vi "VSI Settings Dialog.vi"(8 "error in (no error)":errorcluster, 11 "Ctrl settings in":T1={"FSM status"=enum."Running", "Ctrl bypass"=FALSE, "PID Control"={"Ref_val"=0.0, "Kp"=0.0, "Ti"=0.0, "Td"=16.0, "Out_min"=0.0, "Out_max"=0.0}, "3rd Harmonic"=FALSE, "Output enable"=FALSE, "Phase DBG"=0}) -> (0 "error out":errorcluster, 1 "Cancelled?":bool, 2 "UI Refresh Needed?":bool, 3 "Ctrl settings out":T1={"FSM status"=enum."Running", "Ctrl bypass"=FALSE, "PID Control"={"Ref_val"=0.0, "Kp"=0.0, "Ti"=0.0, "Td"=6.0, "Out_min"=0.0, "Out_max"=0.0}, "3rd Harmonic"=FALSE, "Output enable"=FALSE, "Phase DBG"=0})   [LabVIEW 2015, in "Settings.lvlib"]
doc: "Dialog for selecting user specified settings."
uses:
  Settings.lvlib
  VSI Control settings.ctl
  PID Compensator.ctl
panel:
  in  "Phase DBG":u32=2147 format="%04x"
  in  "Kd":sgl=0.01 caption="Td"
  in  "Ref":sgl=26.0 caption="Vref"
  in  "Ctrl byp":bool caption="Bypass (Ref to Vea)"
  in  "Lim":sgl=250.0 caption="+/- Lim"
  in  "Kp":sgl=100.0
  in  "Ki2":sgl=0.01 caption="Ti"
  in  "3rd harm":bool caption="Third harmonic inj."
  in  "Driver ena":bool=TRUE caption="Driver enable"
  in  "Cancel Button":bool
  in  "Apply Button":bool
  # "Non visible portion of dialog (needed for connector pane)."
  # "da"
  # "db"
  # "dc"
  # "VLa"
  # "VLb"
  # "VLc"
  # "VSI Control"
  # "PWM Generation"
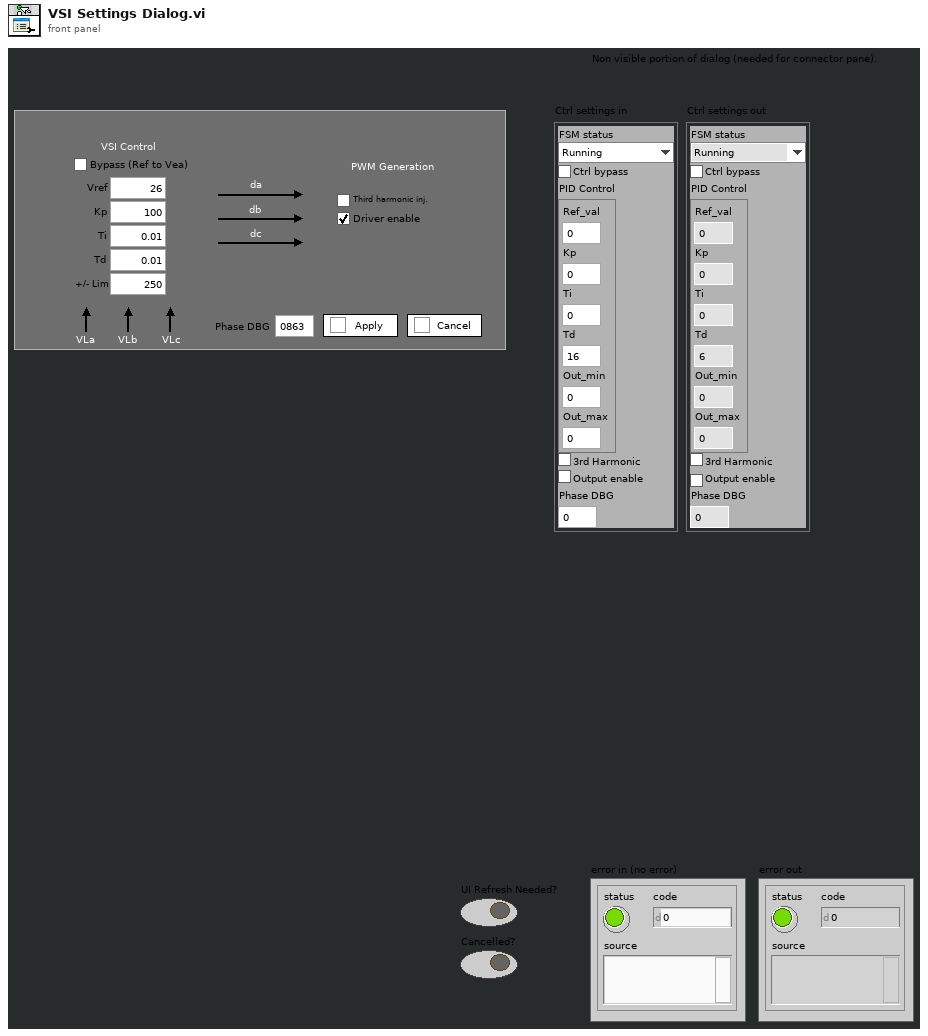
[diagram p1: front panel]
types:
  T1 = typedef "Settings.lvlib/VSI Control settings.ctl" = cluster{"FSM status":enum8{"Stopped", "Running"}, "Ctrl bypass":bool, "PID Control":T2, "3rd Harmonic":bool, "Output enable":bool, "Phase DBG":u32}
  T2 = typedef "Settings.lvlib/PID Compensator.ctl" = cluster{"Ref_val":sgl, "Kp":sgl, "Ti":sgl, "Td":sgl, "Out_min":sgl, "Out_max":sgl}
  T3 = enum8{"Enabled", "Disabled", "Disabled and Grayed Out"}
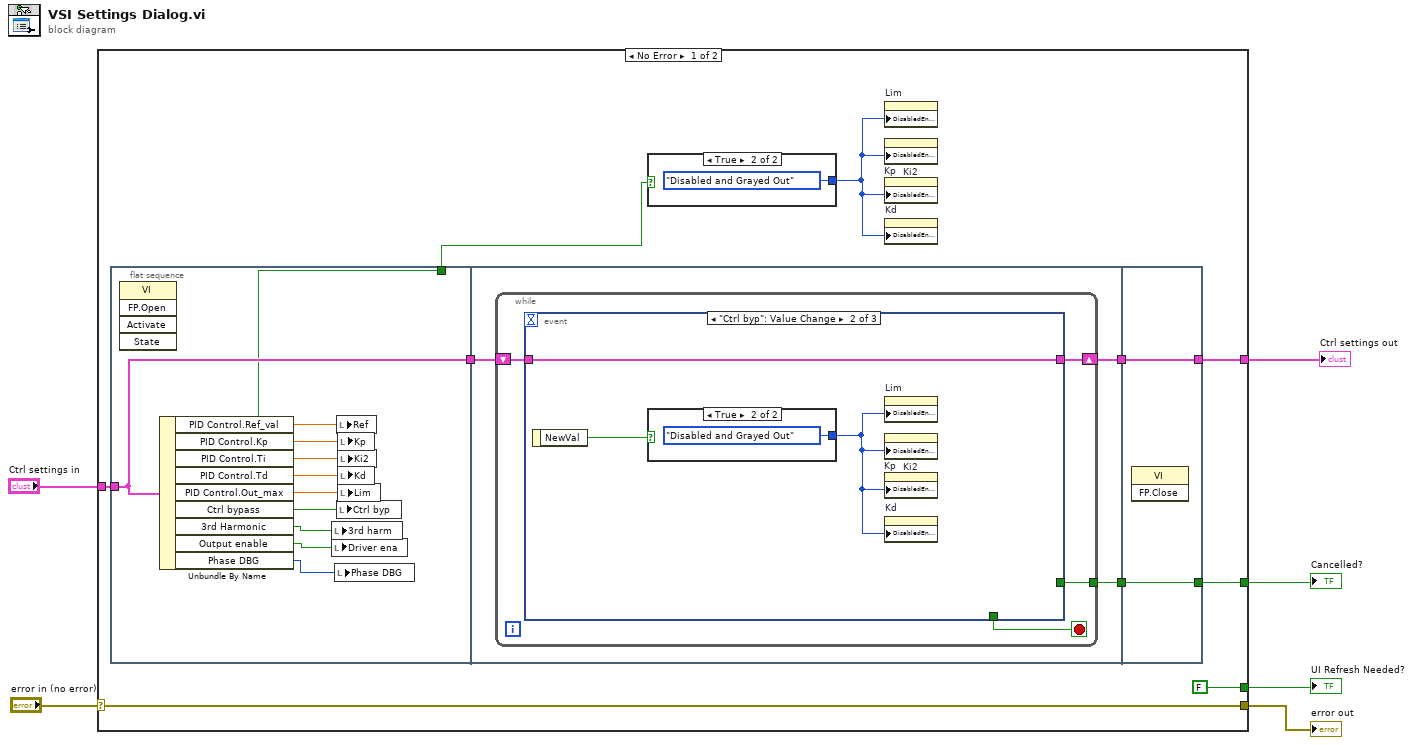
[diagram p0: block diagram]
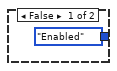
[diagram p2: hidden frame]
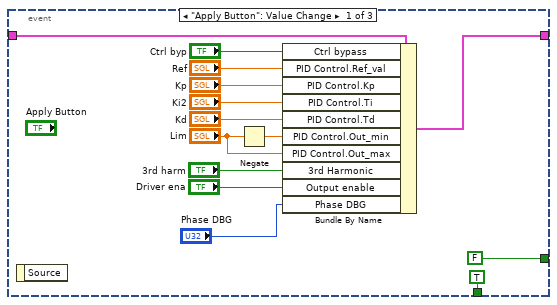
[diagram p3: hidden frame]
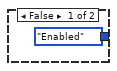
[diagram p4: hidden frame]
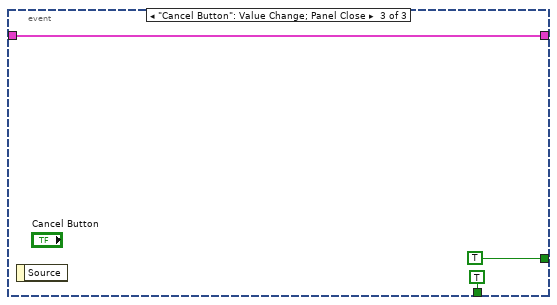
[diagram p5: hidden frame]
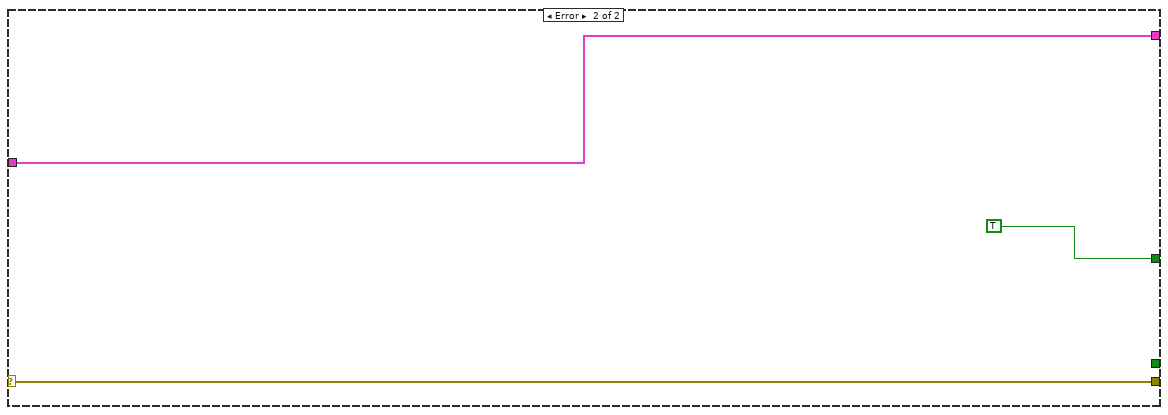
[diagram p6: hidden frame]
diagram:
  n1 = case shown="No Error" "error in (no error)" {
    selector: "error in (no error)" -> [w16 w62]
    tunnel: [w16 w62] -> w5
    tunnel: "Ctrl settings in" -> [w12 w61]
    tunnel: [w13 w61] -> w2
    tunnel: [FALSE ("UI Refresh Needed?") _] -> w4
    tunnel: [w14 TRUE ("UI Refresh Needed?")] -> w3
    frame No Error {
      n2 = flat-sequence {
        tunnel: w12 -> [w26]
        tunnel: [w26] -> w9
        tunnel: [w21] -> w8
        tunnel: [w31] -> w11
        tunnel: [w30] -> w10
        tunnel: w9 -> [w29]
        tunnel: [w58] -> w13
        tunnel: [w59] -> w14
        tunnel: w11 -> [w59]
        tunnel: w10 -> [w58]
        frame #0 {
          n3 = invoke class="VI" method="FP.Open"() -> ()  [unwired: 5 in, 5 out]
          n4 = Unbundle By Name(w26) -> ("PID Control.Ref_val"=w25:sgl, "PID Control.Kp"=w23:sgl, "PID Control.Ti"=w24:sgl, "PID Control.Td"=w20:sgl, "PID Control.Out_max"=w22:sgl, "Ctrl bypass"=w21:bool, "3rd Harmonic"=w28:bool, "Output enable"=w27:bool, "Phase DBG"=w19:u32)
          n5 = local write "3rd harm"(w28) -> ()
          n6 = local write "Driver ena"(w27) -> ()
          n7 = local write "Phase DBG"(w19) -> ()
          n8 = local write "Ref"(w25) -> ()
          n9 = local write "Ctrl byp"(w21) -> ()
          n10 = local write "Kp"(w23) -> ()
          n11 = local write "Ki2"(w24) -> ()
          n12 = local write "Kd"(w20) -> ()
          n13 = local write "Lim"(w22) -> ()
        }
        frame #1 {
          n14 = while {
            tunnel: [w35] -> w31
            shift-right: [w34] -> w30
            shift-left: w29 -> [w33]
            stop <- w32 stop-if-true
            n15 = event shown="[1] \"Ctrl byp\": Value Change" {
              selector: _ -> [_ _ _]
              dyn-events: _ -> [_ _ _]
              timeout: _ -> [_ _ _]
              tunnel: [w47 w52 w57] -> w34
              tunnel: w33 -> [w48 w52 w57]
              tunnel: [FALSE ("UI Refresh Needed?") _ TRUE ("UI Refresh Needed?")] -> w35
              tunnel: [TRUE ("UI Refresh Needed?") _ TRUE ("UI Refresh Needed?")] -> w32
              event "Apply Button": Value Change {
                n16 = event-data() -> ()  [unwired: 1 in, 1 out]
                n17 = Negate(x="Lim") -> (-x=w43:sgl)
                n18 = Bundle By Name(cluster=w48, "Ctrl bypass"="Ctrl byp", "PID Control.Ref_val"="Ref", "PID Control.Kp"="Kp", "PID Control.Ti"="Ki2", "PID Control.Td"="Kd", "PID Control.Out_min"=w43, "PID Control.Out_max"="Lim", "3rd Harmonic"="3rd harm", "Output enable"="Driver ena", "Phase DBG"="Phase DBG") -> (w47:T1)
              }
              event "Ctrl byp": Value Change {
                n19 = event-data() -> ("NewVal"=w51:bool)  [unwired: 1 in]
                n20 = case shown="True" w51 {
                  tunnel: [T3."Enabled" ("Disabled") T3."Disabled and Grayed Out" ("Disabled")] -> w50
                  frame False {
                  }
                  frame True {
                  }
                }
                n21 = property on="Lim" class="DigNum (strict)"("DisabledEnum"=w50) -> ()  [unwired: 2 in, 2 out]
                n22 = property on="Ki2" class="DigNum (strict)"("DisabledEnum"=w50) -> ()  [unwired: 2 in, 2 out]
                n23 = property on="Kp" class="DigNum (strict)"("DisabledEnum"=w50) -> ()  [unwired: 2 in, 2 out]
                n24 = property on="Kd" class="DigNum (strict)"("DisabledEnum"=w50) -> ()  [unwired: 2 in, 2 out]
              }
              event "Cancel Button": Value Change; Panel Close {
                n25 = event-data() -> ()  [unwired: 1 in, 1 out]
              }
            }
          }
        }
        frame #2 {
          n26 = invoke class="VI" method="FP.Close"() -> ()  [unwired: 3 in, 3 out]
        }
      }
      n27 = case shown="True" w8 {
        tunnel: [T3."Enabled" ("Disabled") T3."Disabled and Grayed Out" ("Disabled")] -> w7
        frame False {
        }
        frame True {
        }
      }
      n28 = property on="Lim" class="DigNum (strict)"("DisabledEnum"=w7) -> ()  [unwired: 2 in, 2 out]
      n29 = property on="Ki2" class="DigNum (strict)"("DisabledEnum"=w7) -> ()  [unwired: 2 in, 2 out]
      n30 = property on="Kp" class="DigNum (strict)"("DisabledEnum"=w7) -> ()  [unwired: 2 in, 2 out]
      n31 = property on="Kd" class="DigNum (strict)"("DisabledEnum"=w7) -> ()  [unwired: 2 in, 2 out]
    }
    frame Error {
    }
  }
  "UI Refresh Needed?" <- w4
  "error out" <- w5
  "Cancelled?" <- w3
  "Ctrl settings out" <- w2
